vi "setMeasurement.vi"(8 "error in (no error)":errorcluster, 9 "conversion":T1, 10 "measurement":T2, 11 "Instrument.VSource in":refnum<class "Instrument.VNA.lvclass">) -> (0 "error out":errorcluster, 3 "Instrument.VSource out":refnum<class "Instrument.VNA.lvclass">)   [LabVIEW 2019, in "Instrument.VNA.lvclass"]
uses:
  Instrument.VNA.lvclass
  Typedefs/Measurement--enum.ctl
  Typedefs/Conversion--enum.ctl
  Typedefs/setMeasurement--cluster.ctl
  Typedefs/VNA.Commands--Enum.ctl
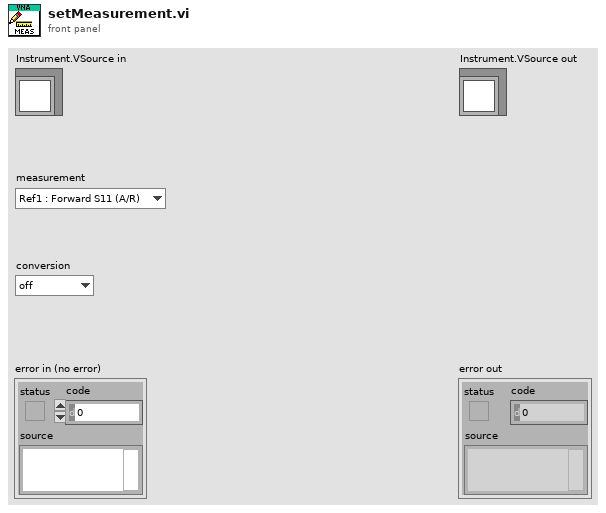
[diagram p1: front panel]
types:
  T1 = typedef "Instrument.VNA.lvclass/Conversion--enum.ctl" = enum16{"off", "Z: Ref1", "Z: Trans", "Y: Ref1", "Y: Trans", "1/S"}
  T2 = typedef "Instrument.VNA.lvclass/Measurement--enum.ctl" = enum16{"Ref1 : Forward S11 (A/R)", "Trans: Forward S21 (B/R)", "Trans: Reverse S12 (A/R)", "Ref1: Reverse S22 (B/R)", "Analog In, AUX input", "A/R", "B/R", "A/B", "A", "B", "R"}
  T3 = typedef "Instrument.VNA.lvclass/VNA.Commands--Enum.ctl" = enum16{"getData", "setAverage", "setFormat", "setMeasurement", "setPower", "setSweep"}
  T4 = typedef "Instrument.VNA.lvclass/setMeasurement--cluster.ctl" = cluster{"measurement":T2, "conversion":T1}
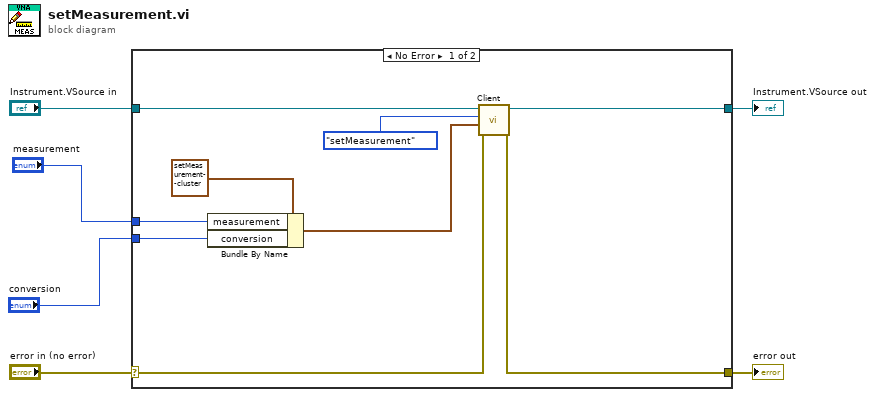
[diagram p0: block diagram]
diagram:
  n1 = case shown="No Error" "error in (no error)" {
    selector: "error in (no error)" -> [w8 w17]
    tunnel: [w13 w17] -> w6
    tunnel: [w14 w16] -> w4
    tunnel: "Instrument.VSource in" -> [w9 w16]
    tunnel: "measurement" -> [w11 _]
    tunnel: "conversion" -> [w10 _]
    frame No Error {
      n2 = Bundle By Name(cluster=T4 {"measurement"=enum."Ref1 : Forward S11 (A/R)", "conversion"=enum."off"} ("seConversion"), "measurement"=w11, "conversion"=w10) -> (w15:T4)
      n3 = call-dynamic "Client.vi"("error in (no error)"=w8, "Data in"=w15, "Command in"=VNA.Commands--Enum."setMeasurement" ("Commands"), "Instrument in"=w9) -> ("error out"=w13:errorcluster, "Instrument out"=w14:refnum<class "Instrument.VNA.lvclass">)  [unwired: 4 in, 2 out]
    }
    frame Error {
    }
  }
  "error out" <- w6
  "Instrument.VSource out" <- w4
